vi "Remove Item.vi"(8 "error in (no error)":errorcluster, 9 "Delete Children":bool=TRUE, 10 "Tag In":string, 11 "Tree in":refnum<class "Tree.lvclass">) -> (0 "error out":errorcluster, 3 "Tree out":refnum<class "Tree.lvclass">)   [LabVIEW 2019, in "Tree.lvclass"]
uses:
  Tree.lvclass
  Tree.lvclass/Tree.ctl
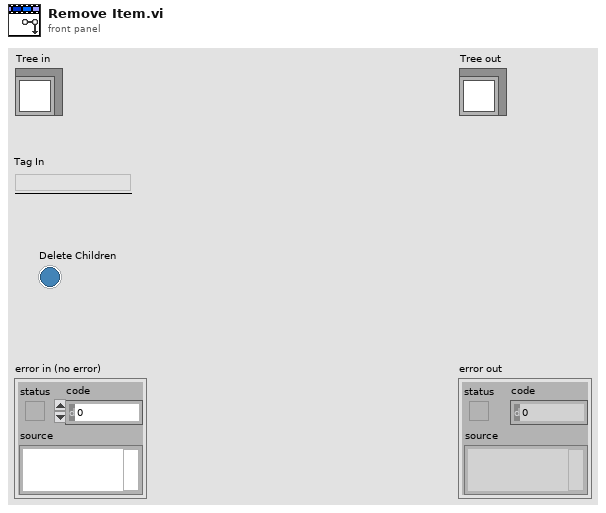
[diagram p1: front panel]
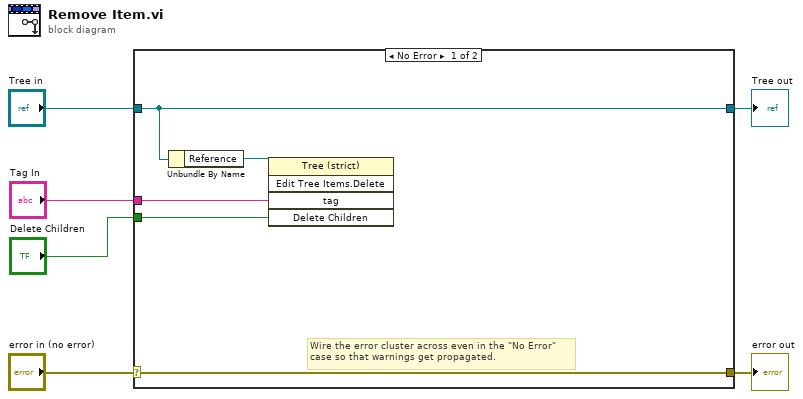
[diagram p0: block diagram]
diagram:
  n1 = case shown="No Error" "error in (no error)" {
    selector: "error in (no error)" -> [w11 w13]
    tunnel: [w11 w13] -> w5
    tunnel: [w10 w12] -> w3
    tunnel: "Tree in" -> [w10 w12]
    tunnel: "Tag In" -> [w8 _]
    tunnel: "Delete Children" -> [w7 _]
    frame No Error {
      # "Wire the error cluster across even in the \"No Error\"\ncase so that warnings get propagated."
      n2 = Unbundle By Name(w10) -> ("Reference"=w9:refnum<vi>)
      n3 = invoke class="Tree (strict)" method="Edit Tree Items.Delete"(reference=w9, "tag"=w8, "Delete Children"=w7) -> ()  [unwired: 2 in, 5 out]
    }
    frame Error {
    }
  }
  "error out" <- w5
  "Tree out" <- w3
